vi "CP1540 Sample.vi"() -> ()   [LabVIEW 2011]
uses:
  Konvolucio MCAN120803 Adapter/Konvolucio MCAN120803 Adapter Class.lvclass
  National Instruments USB-8473 Adapter/National Instruments USB-8473 Adapter Class.lvclass
  Generic CAN Adapter/GenericCanAdapterClass.lvclass
  <vilib>/Utility/miscctls.llb/LVRowAndColumnUnsignedTypeDef.ctl
panel:
  in  "buttonClear":bool
  in  "buttonSave":bool
  in  "buttonScroll":bool
  out "Table Control":string[][](table)
  in  "button_LED_0C42":bool
  in  "button_Stop":bool
  in  "button_Pause":bool
  in  "button_Play":bool
  out "indicatorOpen":bool
  in  "comboInstance":i32(ring) items=["3870366F3133"]
  in  "comboTypes":i32(ring) items=["Generic", "Konvolucio MCAN120803 Adapter", "National Instruments USB-8473 Adapter"]
  # "Type"
  # "Instance"
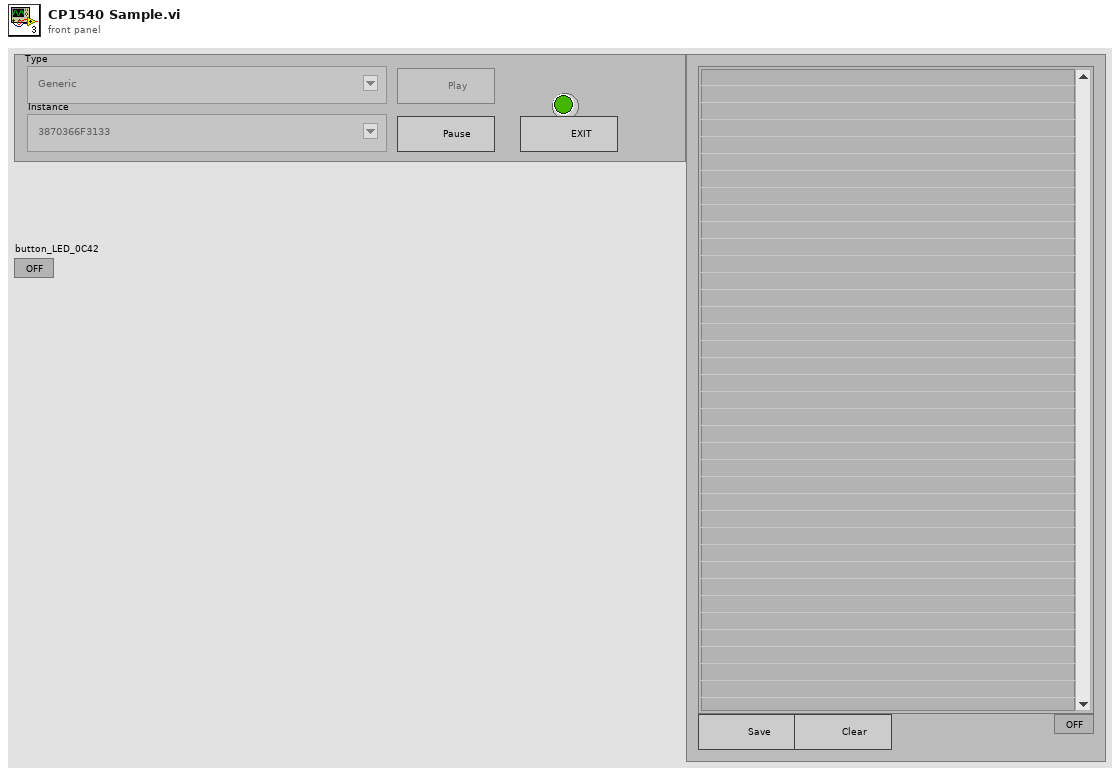
[diagram p1: front panel]
types:
  T1 = typedef "LVRowAndColumnUnsignedTypeDef.ctl" = cluster{"Row":u32, "Column":u32}
  T2 = enum8{"Enabled", "Disabled", "Disabled and Grayed Out"}
  T3 = enum16{"open", "replace", "create", "open or create", "replace or create", "replace or create with confirmation"}
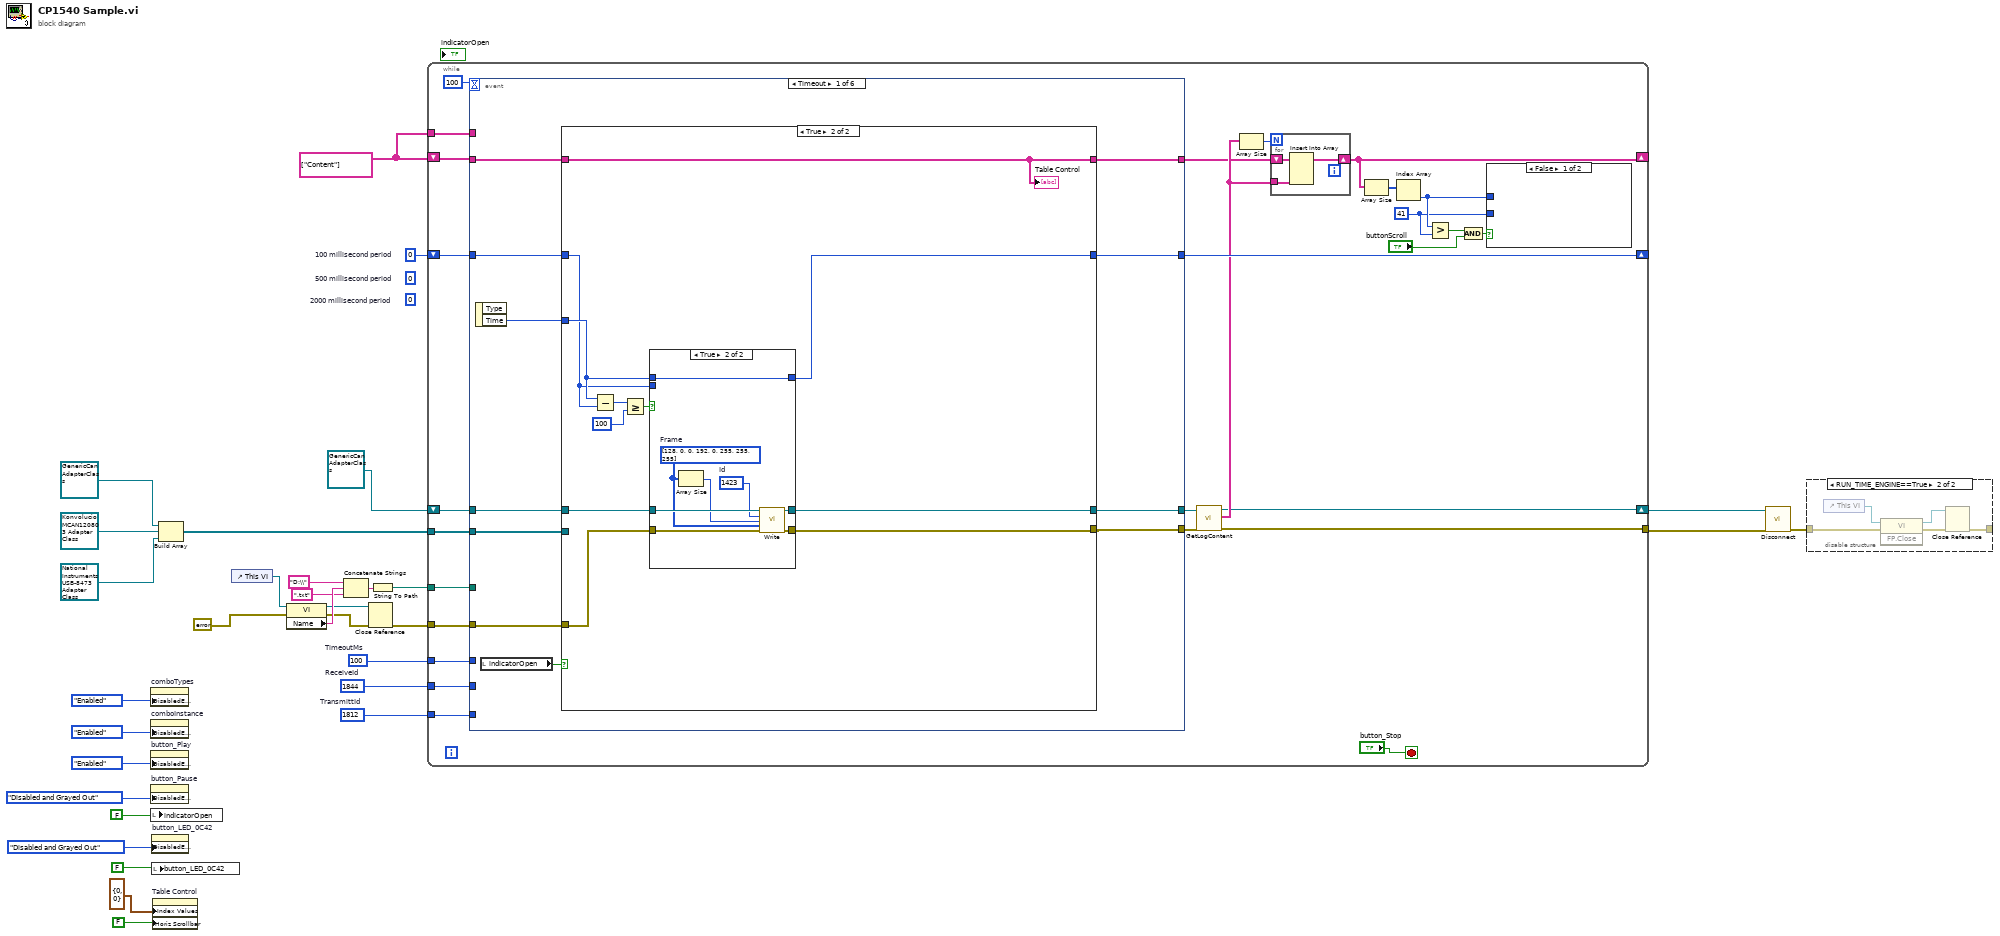
[diagram p0: block diagram]
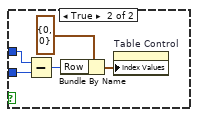
[diagram p3: hidden frame]
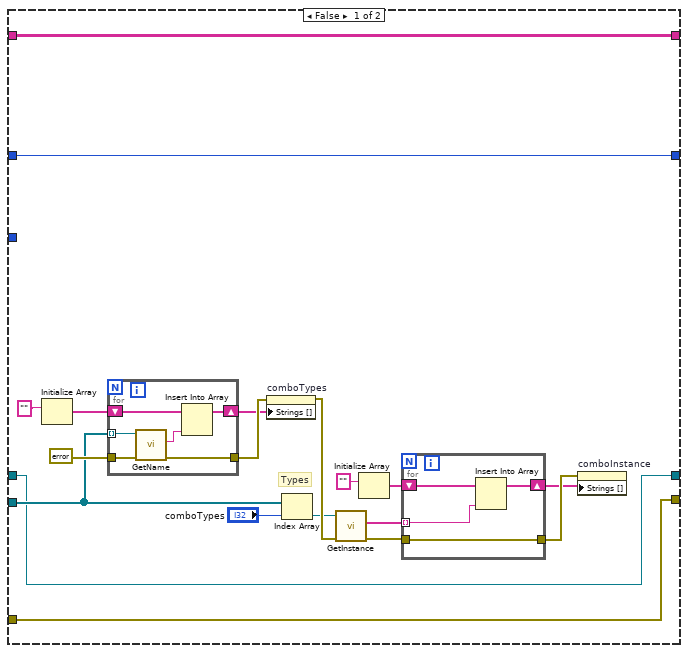
[diagram p4: hidden frame]
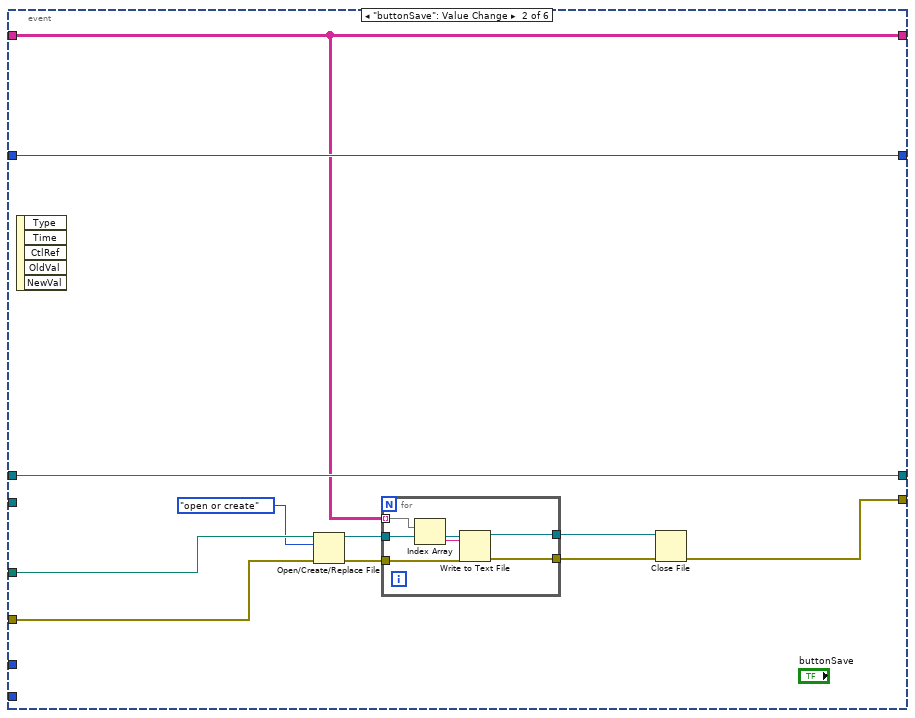
[diagram p6: hidden frame]
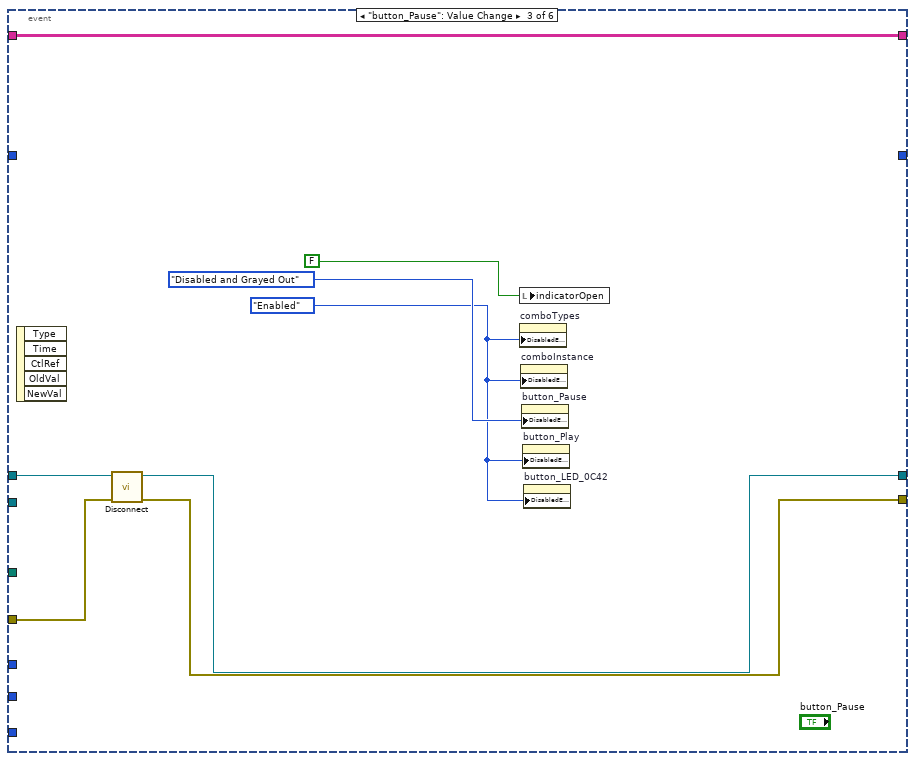
[diagram p7: hidden frame]
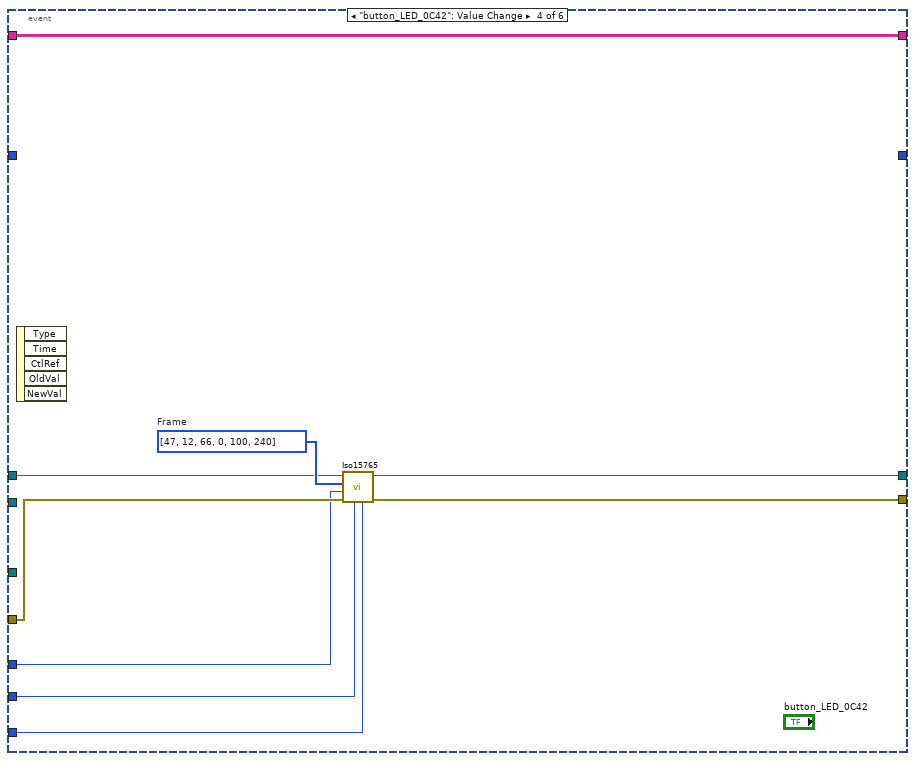
[diagram p8: hidden frame]
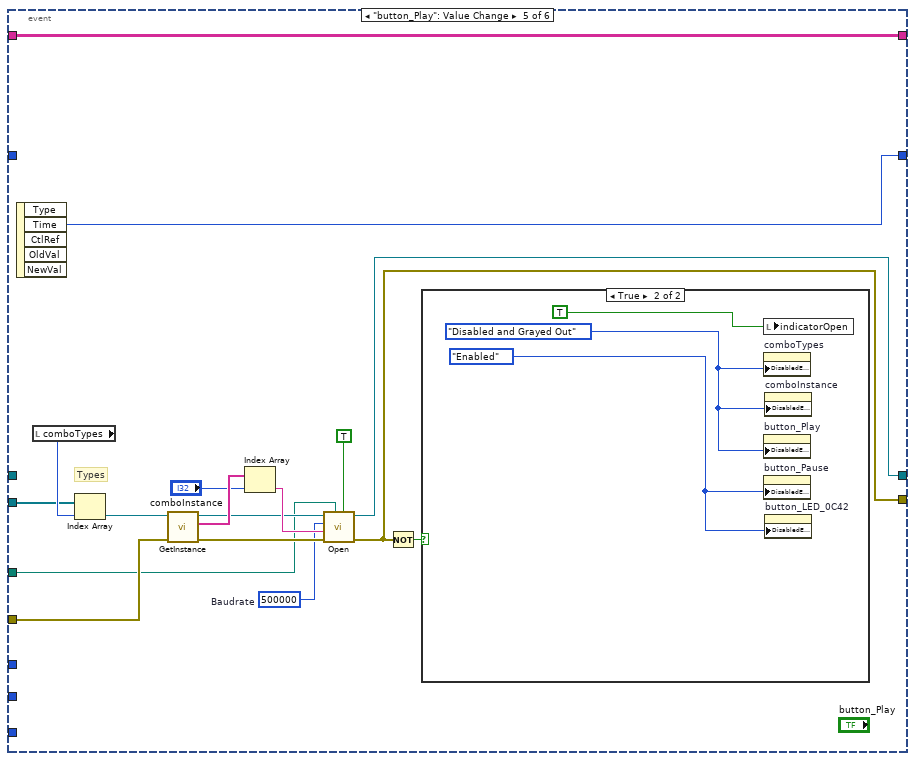
[diagram p9: hidden frame]
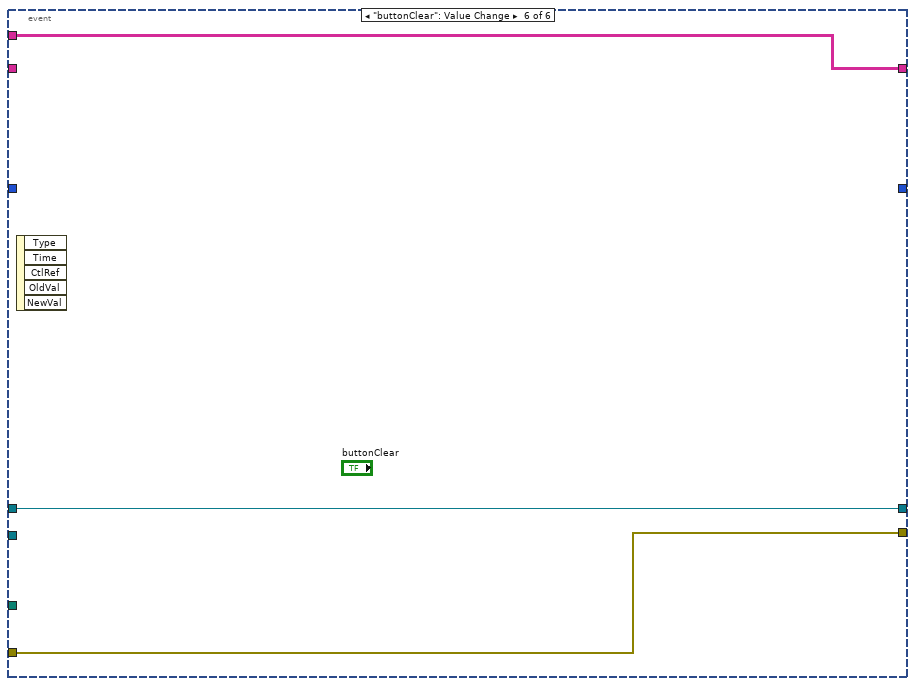
[diagram p11: hidden frame]
diagram:
  w1 = string[][] [["Content"]] ("Table Control 3")
  w6 = u32 100  # TimeoutMs
  w7 = u32 1844  # ReceiveId
  w8 = u32 1812  # TransmittId
  (unwired) u32 0  # 2000 millisecond period
  (unwired) u32 0  # 500 millisecond period
  w11 = u32 0  # 100 millisecond period
  n1 = property on="comboTypes" class="Ring (strict)"("DisabledEnum"=T2."Enabled" ("Disabled")) -> ()  [unwired: 2 in, 2 out]
  n2 = property on="comboInstance" class="Ring (strict)"("DisabledEnum"=T2."Enabled" ("Disabled")) -> ()  [unwired: 2 in, 2 out]
  n3 = property on="button_Play" class="Bool"("DisabledEnum"=T2."Enabled" ("Disabled")) -> ()  [unwired: 2 in, 2 out]
  n4 = property on="button_Pause" class="Bool"("DisabledEnum"=T2."Disabled and Grayed Out" ("Disabled")) -> ()  [unwired: 2 in, 2 out]
  n5 = local write "indicatorOpen"(FALSE ("indicatorOpen")) -> ()
  n6 = property on="button_LED_0C42" class="Bool (strict)"("DisabledEnum"=T2."Disabled and Grayed Out" ("Disabled")) -> ()  [unwired: 2 in, 2 out]
  n7 = local write "button_LED_0C42"(FALSE ("button_LED_0C42")) -> ()
  n8 = property on="Table Control" class="Tbl (strict)"("Index Values"=T1 {"Row"=0, "Column"=0}, "Horiz Scrollbar"=FALSE ("Visible Items:Horizontal Scrollbar Visible")) -> ()  [unwired: 2 in, 2 out]
  n9 = Build Array(refnum<class "GenericCanAdapterClass.lvclass"> refnum ("GenericCanAdapterClass.lvclass"), refnum<class "Konvolucio MCAN120803 Adapter Class.lvclass"> refnum ("Konvolucio MCAN120803 Adapter Class.lvclass"), refnum<class "National Instruments USB-8473 Adapter Class.lvclass"> refnum ("National Instruments USB-8473 Adapter Class.lvclass")) -> (w28:refnum<class "GenericCanAdapterClass.lvclass">[])
  n10 = control-ref of="This VI"() -> (w27:refnum<vi>)
  n11 = property class="VI"(reference=w27, error in=errorcluster {"status"=FALSE, "code"=0, "source"=""} ("error in (no error)")) -> (reference out=w22:refnum<vi>, error out=w21:errorcluster, "Name"=w25:string)
  n12 = Concatenate Strings("D:\\" ("VI Name"), w25, ".txt" ("string")) -> (w23:string)
  n13 = Close Reference(reference=w22, error in (no error)=w21) -> (error out=w20:errorcluster)
  n14 = String To Path(string=w23) -> (path=w18:path)
  n15 = while {
    tunnel: w28 -> [w59]
    tunnel: w20 -> [w56]
    tunnel: w18 -> [w55]
    tunnel: [w37] -> w3
    shift-right: [w52] -> _
    shift-left: w11 -> [w53]
    tunnel: w8 -> [w51]
    tunnel: w7 -> [w50]
    tunnel: w6 -> [w49]
    shift-right: [w34] -> _
    shift-left: w1 -> [w48]
    shift-right: [w36] -> w2
    shift-left: refnum<class "GenericCanAdapterClass.lvclass"> refnum ("GenericCanAdapterClass out") -> [w54]
    tunnel: w1 -> [w35]
    stop <- "button_Stop" stop-if-true
    w42 = 41 ("y")
    n16 = event shown="[0] Timeout" {
      selector: _ -> [_ _ _ _ _ _]
      dyn-events: _ -> [_ _ _ _ _ _]
      timeout: 100 -> [_ _ _ _ _ _]
      tunnel: w59 -> [w77 _ _ _ w178 _]
      tunnel: w56 -> [w76 w133 w153 w161 w177 w185]
      tunnel: w55 -> [_ w134 _ _ w167 _]
      tunnel: [w70 w132 w150 w160 w169 w185] -> w38
      tunnel: [w71 w139 w149 w159 w164 w186] -> w39
      tunnel: w54 -> [w73 w139 w154 w162 _ w186]
      tunnel: w53 -> [w74 w140 _ _ _ _]
      tunnel: [w72 w140 _ _ w166 _] -> w52
      tunnel: w51 -> [_ _ _ w158 _ _]
      tunnel: w50 -> [_ _ _ w157 _ _]
      tunnel: w49 -> [_ _ _ w156 _ _]
      tunnel: w48 -> [w68 w130 w147 w155 w165 _]
      tunnel: [w69 w130 w147 w155 w165 w184] -> w33
      tunnel: w35 -> [_ _ _ _ _ w184]
      event Timeout {
        n17 = event-data() -> ("Time"=w75:u32)  [unwired: 1 in, 1 out]
        n18 = local read "indicatorOpen"() -> (w78:bool)
        n19 = case shown="True" w78 {
          tunnel: w77 -> [w83 _]
          tunnel: w76 -> [w80 w113]
          tunnel: w75 -> [_ w111]
          tunnel: w74 -> [w81 w110]
          tunnel: w73 -> [w82 w115]
          tunnel: [w82 w114] -> w71
          tunnel: [w81 w112] -> w72
          tunnel: [w80 w109] -> w70
          tunnel: [w79 w108] -> w69
          tunnel: w68 -> [w79 w108]
          frame False {
            # "Types"
            n20 = Initialize Array("") -> (w85:string[])  [unwired: 1 in]
            n21 = for {
              shift-right: [w107] -> w87
              shift-left: w85 -> [w106]
              tunnel: w83 -> [w105] mode=indexing
              tunnel: errorcluster {"status"=FALSE, "code"=0, "source"=""} ("error in (no error)") -> [w103]
              tunnel: [w102] -> w88
              n22 = call-dynamic "GetName.vi"("error in (no error)"=w103, "GenericCanAdapterClass in"=w105) -> ("error out"=w102:errorcluster, "Value"=w104:string)  [unwired: 7 in, 1 out]
              n23 = Insert Into Array(array=w106, new element=w104) -> (w107:string[])  [unwired: 1 in]
            }
            n24 = property on="comboTypes" class="Ring (strict)"(error in=w88, "Strings []"=w87) -> (error out=w94:errorcluster)  [unwired: 1 in, 1 out]
            n25 = Index Array(array=w83, index="comboTypes") -> (element=w93:refnum<class "GenericCanAdapterClass.lvclass">)
            n26 = call-dynamic "GetInstance.vi"("error in (no error)"=w94, "GenericCanAdapterClass in"=w93) -> ("error out"=w95:errorcluster, "Values"=w96:string[])  [unwired: 7 in, 1 out]
            n27 = Initialize Array("") -> (w89:string[])  [unwired: 1 in]
            n28 = for {
              shift-right: [w101] -> w91
              shift-left: w89 -> [w100]
              tunnel: [w99] -> w92
              tunnel: w95 -> [w99]
              tunnel: w96 -> [w98] mode=indexing
              n29 = Insert Into Array(array=w100, new element=w98) -> (w101:string[])  [unwired: 1 in]
            }
            n30 = property on="comboInstance" class="Ring (strict)"(error in=w92, "Strings []"=w91) -> ()  [unwired: 1 in, 2 out]
          }
          frame True {
            n31 = Subtract(x=w111, y=w110) -> (x-y=w118:u32)
            n32 = Greater Or Equal?(x=w118, y=u32 100) -> (x >= y?=w116:bool)
            n33 = case shown="True" w116 {
              tunnel: w115 -> [w121 w129]
              tunnel: [w121 w128] -> w114
              tunnel: w113 -> [w120 w127]
              tunnel: [w120 w126] -> w109
              tunnel: [w119 w122] -> w112
              tunnel: w111 -> [_ w122]
              tunnel: w110 -> [w119 _]
              frame False {
              }
              frame True {
                w123 = u32 1423  # Id
                w125 = u8[] [128, 0, 0, 192, 0, 255, 255, 255]  # Frame
                n34 = Array Size(array=w125) -> (size(s)=w124:i32)
                n35 = call-dynamic "Write.vi"("GenericCanAdapterClass in"=w129, "Id"=w123, "DataLength"=w124, "Data"=w125, "error in (no error)"=w127) -> ("GenericCanAdapterClass out"=w128:refnum<class "GenericCanAdapterClass.lvclass">, "error out"=w126:errorcluster)  [unwired: 9 in]
              }
            }
            "Table Control" <- w108
          }
        }
      }
      event "buttonSave": Value Change {
        n36 = event-data() -> ()  [unwired: 1 in, 5 out]
        n37 = Open/Create/Replace File(file path (use dialog)=w134, error in=w133, operation (0:open)=T3."open or create") -> (refnum out=w138:refnum<file>, error out=w137:errorcluster)  [unwired: 3 in, 1 out]
        n38 = for {
          tunnel: w138 -> [w146]
          tunnel: w137 -> [w145]
          tunnel: [w144] -> w136
          tunnel: [w143] -> w135
          tunnel: w130 -> [w142] mode=indexing
          n39 = Index Array(array=w142) -> (element=w141:string)  [unwired: 1 in]
          n40 = Write to Text File(file (use dialog)=w146, text=w141, error in=w145) -> (refnum out=w144:refnum<file>, error out=w143:errorcluster)  [unwired: 1 in, 1 out]
        }
        n41 = Close File(refnum=w136, error in=w135) -> (error out=w132:errorcluster)  [unwired: 1 out]
      }
      event "button_Pause": Value Change {
        w148 = T2."Enabled" ("Disabled")
        n42 = event-data() -> ()  [unwired: 1 in, 5 out]
        n43 = call "Disconnect.vi"("error in (no error)"=w153, "GenericCanAdapterClass in"=w154) -> ("error out"=w150:errorcluster, "GenericCanAdapterClass out"=w149:refnum<class "GenericCanAdapterClass.lvclass">)  [unwired: 7 in]
        n44 = local write "indicatorOpen"(FALSE ("indicatorOpen")) -> ()
        n45 = property on="comboTypes" class="Ring (strict)"("DisabledEnum"=w148) -> ()  [unwired: 2 in, 2 out]
        n46 = property on="comboInstance" class="Ring (strict)"("DisabledEnum"=w148) -> ()  [unwired: 2 in, 2 out]
        n47 = property on="button_Pause" class="Bool"("DisabledEnum"=T2."Disabled and Grayed Out" ("Disabled")) -> ()  [unwired: 2 in, 2 out]
        n48 = property on="button_Play" class="Bool"("DisabledEnum"=w148) -> ()  [unwired: 2 in, 2 out]
        n49 = property on="button_LED_0C42" class="Bool (strict)"("DisabledEnum"=w148) -> ()  [unwired: 2 in, 2 out]
      }
      event "button_LED_0C42": Value Change {
        w163 = u8[] [47, 12, 66, 0, 100, 240]  # Frame
        n50 = event-data() -> ()  [unwired: 1 in, 5 out]
        n51 = call "Iso15765.vi"("TransmittId"=w158, "ReceiveId"=w157, "error in (no error)"=w161, "TimeoutMs"=w156, "Request"=w163, "GenericCanAdapterClass in"=w162) -> ("error out"=w160:errorcluster, "GenericCanAdapterClass out"=w159:refnum<class "GenericCanAdapterClass.lvclass">)  [unwired: 3 in, 1 out]
      }
      event "button_Play": Value Change {
        w171 = u32 500000  # Baudrate
        # "Types"
        n52 = event-data() -> ("Time"=w166:u32)  [unwired: 1 in, 4 out]
        n53 = local read "comboTypes"() -> (w179:i32)
        n54 = Index Array(array=w178, index=w179) -> (element=w180:refnum<class "GenericCanAdapterClass.lvclass">)
        n55 = call-dynamic "GetInstance.vi"("error in (no error)"=w177, "GenericCanAdapterClass in"=w180) -> ("error out"=w174:errorcluster, "Values"=w176:string[], "GenericCanAdapterClass out"=w172:refnum<class "GenericCanAdapterClass.lvclass">)  [unwired: 7 in]
        n56 = Index Array(array=w176, index="comboInstance") -> (element=w173:string)
        n57 = call-dynamic "Open.vi"("LogEnabled"=TRUE, "LogPath"=w167, "error in (no error)"=w174, "Instance"=w173, "BaudRate"=w171, "GenericCanAdapterClass in"=w172) -> ("error out"=w169:errorcluster, "GenericCanAdapterClass out"=w164:refnum<class "GenericCanAdapterClass.lvclass">)  [unwired: 4 in]
        n58 = Not(x=w169) -> (.not. x?=w168:bool)
        n59 = case shown="True" w168 {
          frame False {
          }
          frame True {
            w181 = T2."Enabled" ("Disabled")
            w182 = T2."Disabled and Grayed Out" ("Disabled")
            n60 = local write "indicatorOpen"(TRUE ("indicatorOpen")) -> ()
            n61 = property on="comboTypes" class="Ring (strict)"("DisabledEnum"=w182) -> ()  [unwired: 2 in, 2 out]
            n62 = property on="button_Play" class="Bool"("DisabledEnum"=w182) -> ()  [unwired: 2 in, 2 out]
            n63 = property on="button_Pause" class="Bool"("DisabledEnum"=w181) -> ()  [unwired: 2 in, 2 out]
            n64 = property on="comboInstance" class="Ring (strict)"("DisabledEnum"=w182) -> ()  [unwired: 2 in, 2 out]
            n65 = property on="button_LED_0C42" class="Bool (strict)"("DisabledEnum"=w181) -> ()  [unwired: 2 in, 2 out]
          }
        }
      }
      event "buttonClear": Value Change {
        n66 = event-data() -> ()  [unwired: 1 in, 5 out]
      }
    }
    n67 = call-dynamic "GetLogContent.vi"("error in (no error)"=w38, "GenericCanAdapterClass in"=w39) -> ("error out"=w37:errorcluster, "LogContent"=w40:string[], "GenericCanAdapterClass out"=w36:refnum<class "GenericCanAdapterClass.lvclass">)  [unwired: 7 in]
    n68 = Array Size(array=w40) -> (size(s)=w41:i32)
    n69 = for {
      N: w41 -> [_]
      tunnel: w40 -> [w60]
      shift-right: [w61] -> w34
      shift-left: w33 -> [w62]
      n70 = Insert Into Array(array=w62, new element=w60) -> (w61:string[][])  [unwired: 2 in]
    }
    n71 = Array Size(array=w34) -> (size(s)=w47:i32[])
    n72 = Index Array(array=w47) -> (element=w45:i32)  [unwired: 1 in]
    n73 = Greater?(x=w45, y=w42) -> (0:w44:bool)
    n74 = And(x=w44, y="buttonScroll") -> (x .and. y?=w43:bool)
    n75 = case shown="False" w43 {
      tunnel: w45 -> [_ w67]
      tunnel: w42 -> [_ w63]
      frame False {
      }
      frame True {
        n76 = Subtract(x=w67, y=w63) -> (x-y=w65:i32)
        n77 = Bundle By Name(cluster=T1 {"Row"=0, "Column"=0} ("Index Values"), "Row"=w65) -> (w64:T1)
        n78 = property on="Table Control" class="Tbl (strict)"("Index Values"=w64) -> ()  [unwired: 2 in, 2 out]
      }
    }
  }
  n79 = call "Disconnect.vi"("error in (no error)"=w3, "GenericCanAdapterClass in"=w2) -> ("error out"=w17:errorcluster)  [unwired: 7 in, 1 out]
  n80 = disable-structure shown="RUN_TIME_ENGINE==True" {
    disable-tunnel: w17 -> [w187 w189]
    disable-tunnel: [w187 w188] -> _
    frame condition #0 (active) {
    }
    frame condition #1 {
      n81 = control-ref of="This VI"() -> (w191:refnum<vi>)
      n82 = invoke class="VI" method="FP.Close"(reference=w191, error in=w189) -> (reference out=w190:refnum<vi>, error out=w192:errorcluster)  [unwired: 1 in, 1 out]
      n83 = Close Reference(reference=w190, error in (no error)=w192) -> (error out=w188:errorcluster)
    }
  }
